vi "Remove Node.vi"(7 "Node Path":string, 11 "Tree Map In":T1) -> (0 "Path Invalid":bool, 3 "Tree Map Out":T1, 5 "Removed Paths":set{string}(c389))   [LabVIEW 2021, in "Tree Map.lvlib"]
doc: "Remove a node from the Tree Map. This method is recursive and will remove all children nodes.\n\n<b>Author:</b> Piotr Kruczkowski <PrimaryKey>\n<b>License:</b> NewBSD\n\nCopyright (c) 2019, National Instruments\nAll rights reserved.\n\nRedistribution and use in source and binary forms, with or without\nmodification, are permitted provided that the following conditions are met:\n1. Redistributions of source code must retain the above copyright\n notice, this list of conditions and the following disclaimer.\n2. Redistributions in binary form must reproduce the above copyright\n notice, this list of conditions and the following disclaimer in the\n documentation and/or other materials provided with the distribution.\n3. Neither the name of National Instruments nor the\n names of its contributors may be used to endorse or promote products\n derived from this software without specific prior written permission.\n\nTHIS SOFTWARE IS PROVIDED BY National Instruments ''AS IS'' AND ANY\nEXPRESS OR IMPLIED WARRANTIES, INCLUDING, BUT NOT LIMITED TO, THE IMPLIED\nWARRANTIES OF MERCHANTABILITY AND FITNESS FOR A PARTICULAR PURPOSE ARE\nDISCLAIMED. IN NO EVENT SHALL National Instruments BE LIABLE FOR ANY\nDIRECT, INDIRECT, INCIDENTAL, SPECIAL, EXEMPLARY, OR CONSEQUENTIAL DAMAGES\n(INCLUDING, BUT NOT LIMITED TO, PROCUREMENT OF SUBSTITUTE GOODS OR SERVICES;\nLOSS OF USE, DATA, OR PROFITS; OR BUSINESS INTERRUPTION) HOWEVER CAUSED AND\nON ANY THEORY OF LIABILITY, WHETHER IN CONTRACT, STRICT LIABILITY, OR TORT\n(INCLUDING NEGLIGENCE OR OTHERWISE) ARISING IN ANY WAY OUT OF THE USE OF THIS\nSOFTWARE, EVEN IF ADVISED OF THE POSSIBILITY OF SUCH DAMAGE."
uses:
  <vilib>/National Instruments/Tree Map/Tree Map.lvlib
  <vilib>/National Instruments/Tree Map/Tree Map Data.ctl
  f540c17d-5f24-4b23-b227-3f94d9164d3c.vi
  <vilib>/National Instruments/Tree Map/Utility/Join Strings Tree.vi
  <vilib>/National Instruments/Tree Map/SubVIs/TM Head and Tail.vi
  <vilib>/National Instruments/Tree Map/SubVIs/TM Init and Last.vi
  <vilib>/National Instruments/Tree Map/Utility/Split String Tree.vi
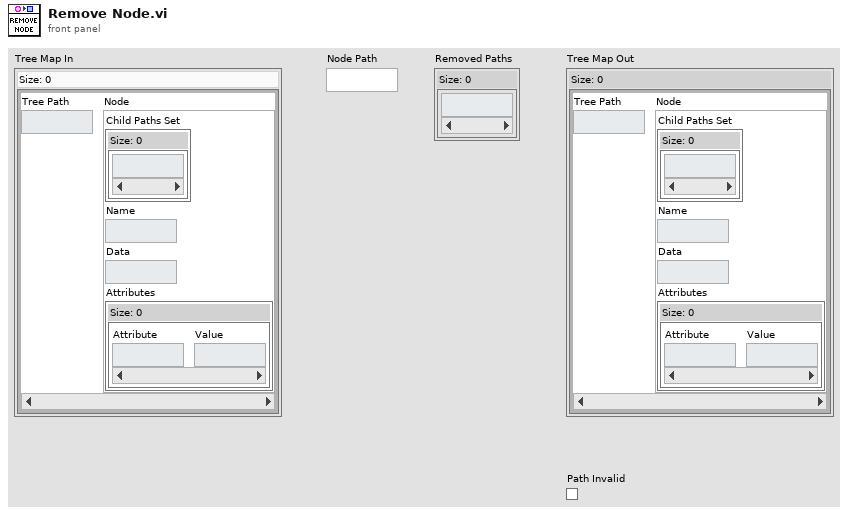
[diagram p1: front panel]
types:
  T1 = typedef "Tree Map.lvlib/Tree Map Data.ctl" = map{string, cluster{"Child Paths Set":set{string}, "Name":string, "Data":string, "Attributes":map{string, string}}}
  T2 = cluster{"Child Paths Set":set{string}, "Name":string, "Data":string, "Attributes":map{string, string}}
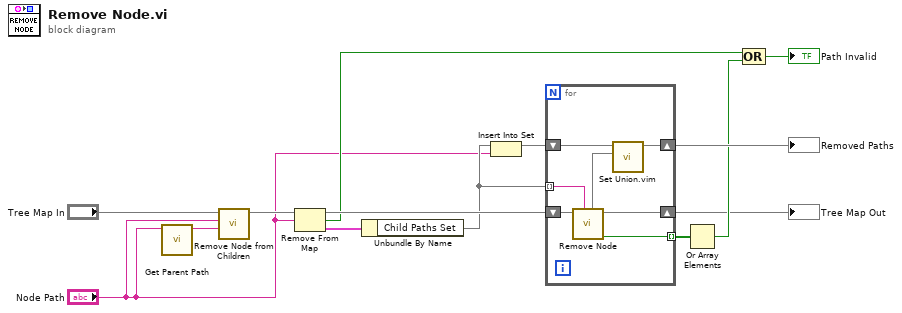
[diagram p0: block diagram]
diagram:
  n1 = call <vilib>:"Get Parent Path.vi"("Node Path"="Node Path") -> ("Parent Path"=w2:string)  [unwired: 8 in, 2 out]
  n2 = call <vilib>:"Remove Node from Children.vi"("Parent Path"=w2, "Node Path In"="Node Path", "Tree Map In"="Tree Map In") -> ("Tree Map Out"=w3:T1)  [unwired: 7 in, 1 out]
  n3 = Remove From Map(10:"Node Path", 11:w3) -> (1:w13:T2, 2:w8:bool, 3:w14:T1)
  n4 = Unbundle By Name(w13) -> ("Child Paths Set"=w6:set{string})
  n5 = Insert Into Set(10:"Node Path", 11:w6) -> (3:w12:set{string})  [unwired: 1 out]
  n6 = for {
    shift-right: [w20] -> w5
    shift-left: w14 -> [w21]
    tunnel: w6 -> [w17] mode=indexing
    shift-right: [w18] -> w11
    shift-left: w12 -> [w19]
    tunnel: [w15] -> w10 mode=indexing
    n7 = call <vilib>:"Remove Node.vi"("Node Path"=w17, "Tree Map In"=w21) -> ("Path Invalid"=w15:bool, "Tree Map Out"=w20:T1, "Removed Paths"=w16:set{string})  [unwired: 7 in]
    n8 = call "Set Union.vim"("set 2"=w16, "set 1"=w19) -> ("union"=w18:set{string})  [unwired: 9 in]
  }
  "Removed Paths" <- w11
  "Tree Map Out" <- w5
  n9 = Or Array Elements(Boolean array=w10) -> (logical OR=w9:bool)
  n10 = Compound Arithmetic op=OR(w8, w9) -> (→"Path Invalid":bool)
